vi "Untitled 1.vi"() -> ()   [LabVIEW 2017]
panel:
  in  "data in":dbl
  out "data out":dbl
  in  "stop":bool
  in  "Variable2":dbl
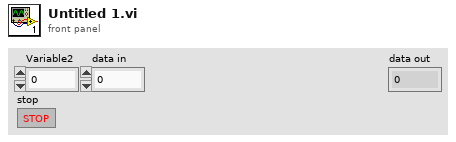
[diagram p1: front panel]
types:
  T1 = cluster{"Read Access":enum8{"Allowed", "Required", "None"}, "Write Access":enum8{"Allowed", "Required", "None"}}
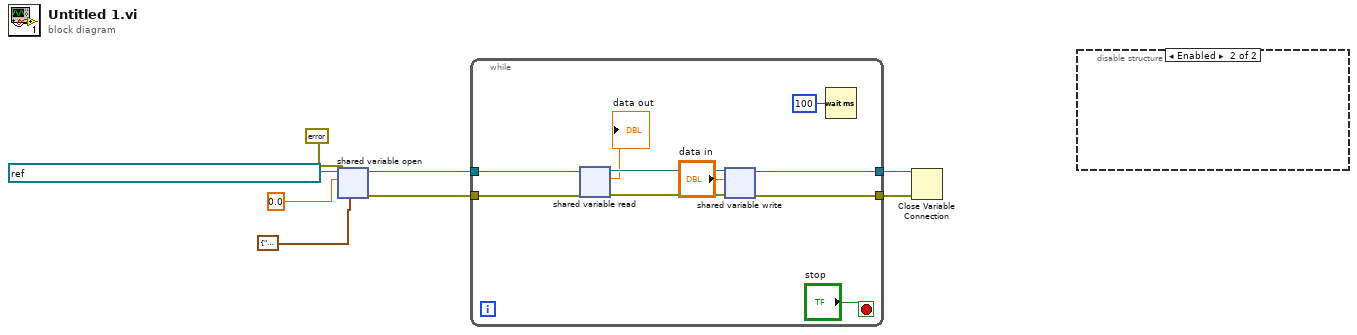
[diagram p0: block diagram]
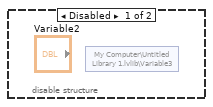
[diagram p2: hidden frame]
diagram:
  n1 = shared-variable-open(refnum<k21> "ni.var.psp://my computer/Untitled Library 1/Variable3" ("shared variable refnum in"), errorcluster {"status"=FALSE, "code"=0, "source"=""} ("error in (no error)"), 0.0, T1 {"Read Access"=enum."Allowed", "Write Access"=enum."Allowed"} ("access")) -> (w7:refnum<k21>, w6:errorcluster)
  n2 = while {
    tunnel: w7 -> [w16]
    tunnel: w6 -> [w15]
    tunnel: [w10] -> w1
    tunnel: [w9] -> w2
    stop <- "stop" stop-if-true
    n3 = shared-variable-read(w16, w15) -> (w14:refnum<k21>, w13:errorcluster, →"data out":dbl)  [unwired: 1 out]
    n4 = shared-variable-write(w14, w13, "data in") -> (w10:refnum<k21>, w9:errorcluster)
    n5 = Wait (ms)(milliseconds to wait=u32 100) -> ()  [unwired: 1 out]
  }
  n6 = Close Variable Connection(8:w2, 11:w1) -> ()  [unwired: 1 out]
  n7 = disable-structure shown="Enabled" {
    frame Disabled {
      n8 = shared-variable "My Computer\\Untitled Library 1.lvlib\\Variable3"() -> ()  [unwired: 2 in, 1 out]
    }
    frame Enabled {
    }
  }
